vi "State Machine.vi"() -> ()   [LabVIEW 2020]
uses:
  enum control.ctl
  <vilib>/Utility/config.llb/NI_LVConfig.lvlib
panel:
  out "Ring":u16(ring)
  out "Time remaning":string
  out "numerator":dbl
  out "Duration of centrifugation":dbl
  out "Duration of rinsing":dbl
  out "Duration of washing":dbl
  out "Spin":dbl(slide) scale=0.0..1200.0
  out "Temperature":dbl(slide) scale=0.0..100.0
  out "Program 4":string
  out "Program 3":string
  out "Program 2":string
  out "Program 1":string
  in  "Stop Button":bool
  out "Lock Button":bool
  in  "Play Button":bool
  in  "Program":u32(knob) max=3 scale=0.0..3.0
  out "Centrifugation":bool
  out "Rinsing":bool
  out "Washing":bool
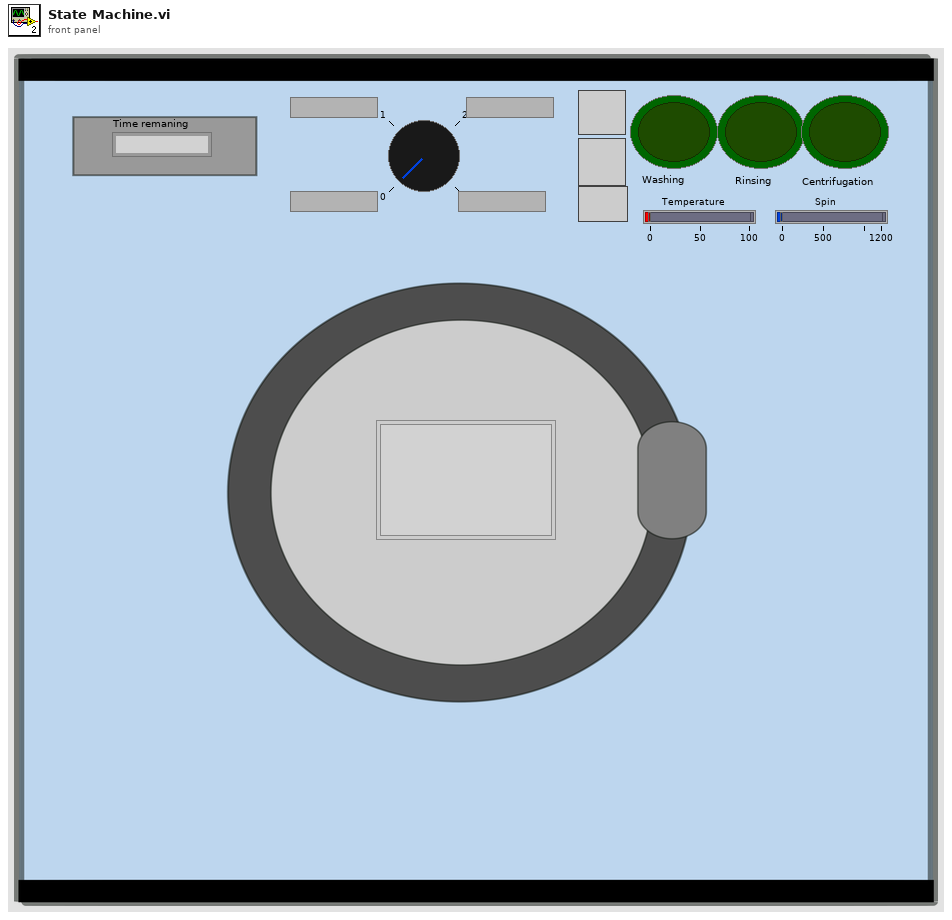
[diagram p1: front panel]
types:
  T1 = cluster{"Results":u32[], "Results":u32[], "Results":u32[], "Results":u32[]}
  T2 = typedef "enum control.ctl" = enum16{"Init", "Which program", "Block", "Washing", "Rinsing", "Centrifugation", "Unblock", "End"}
  T3 = enum8{"Enabled", "Disabled", "Disabled and Grayed Out"}
  T4 = typedef "NI_LVConfig.lvlib/Config Data RefNum.ctl" = refnum<k1>
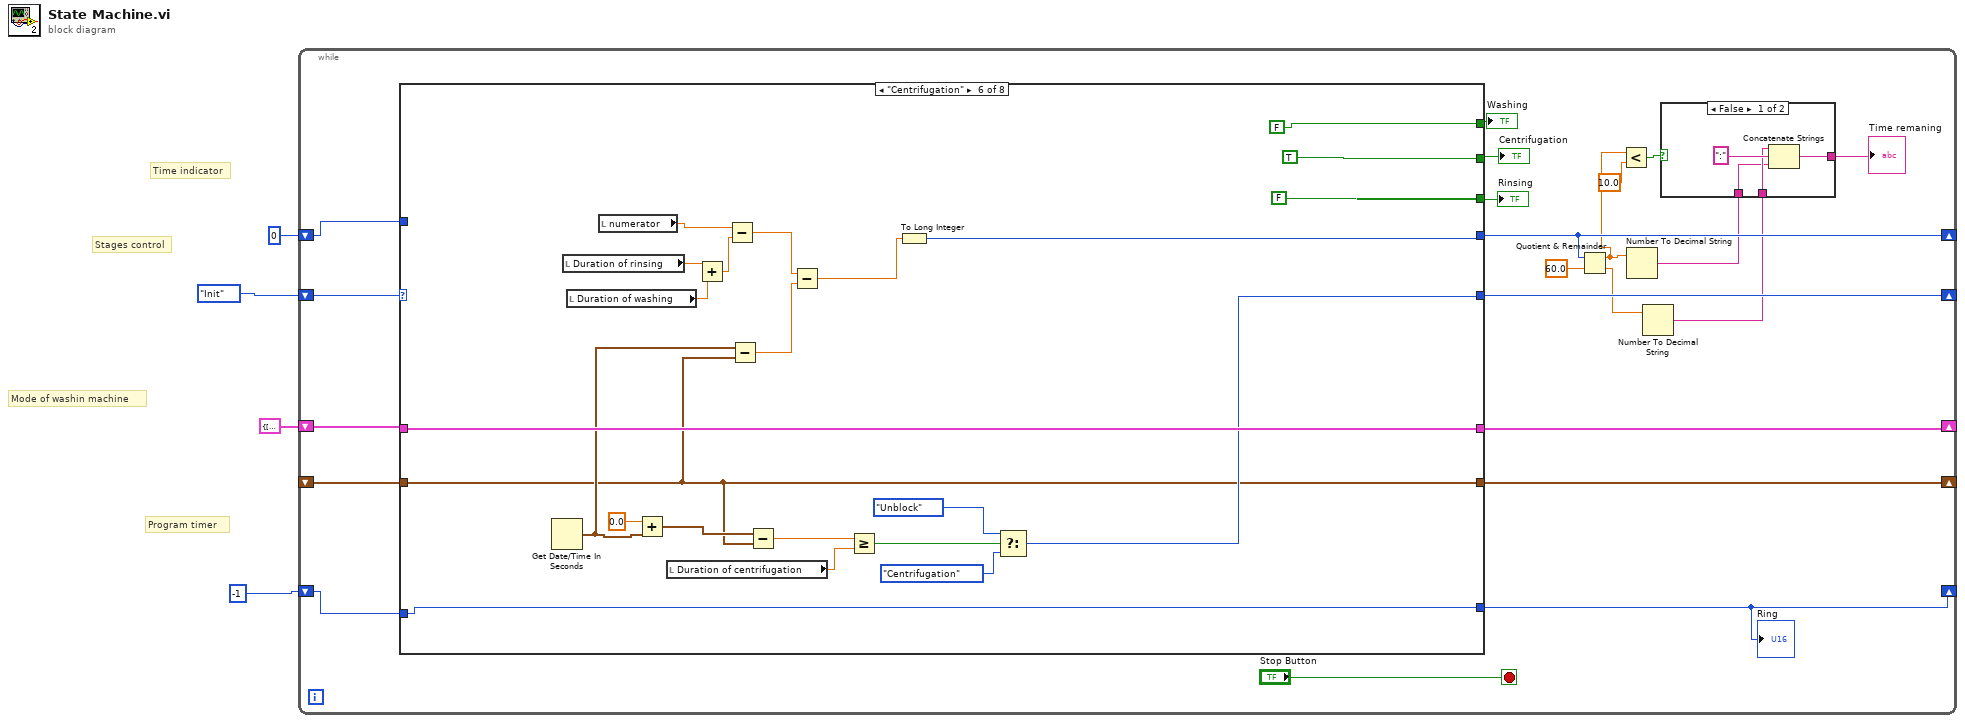
[diagram p0: block diagram]
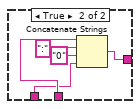
[diagram p2: hidden frame]
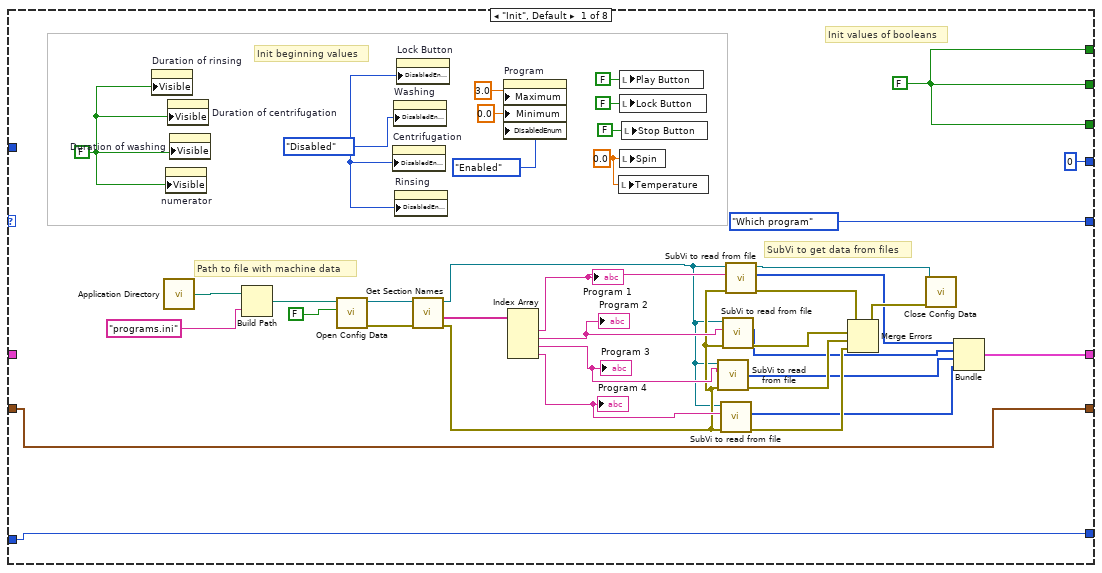
[diagram p3: hidden frame]
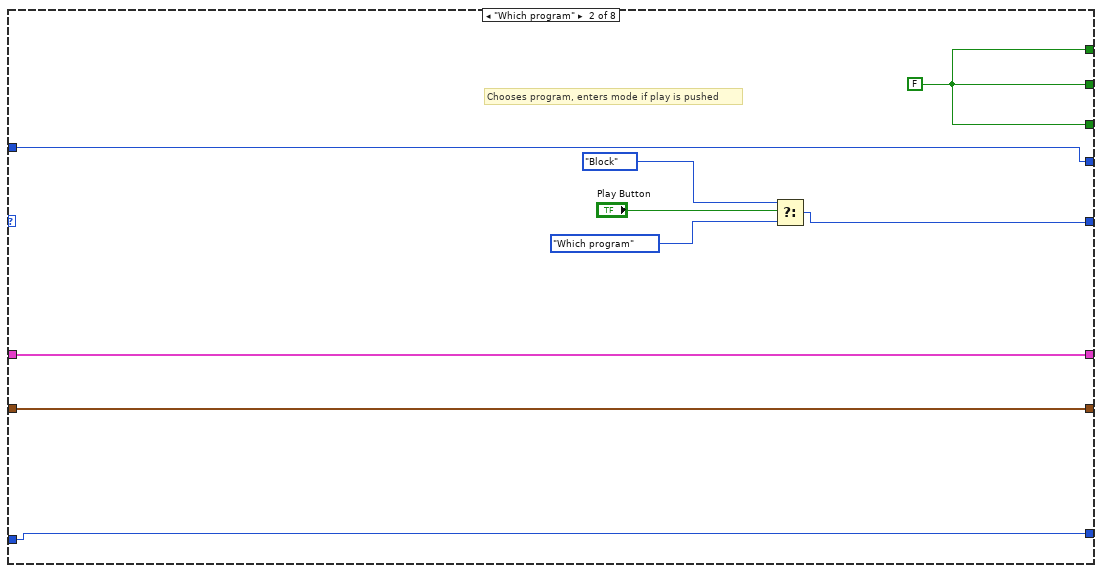
[diagram p4: hidden frame]
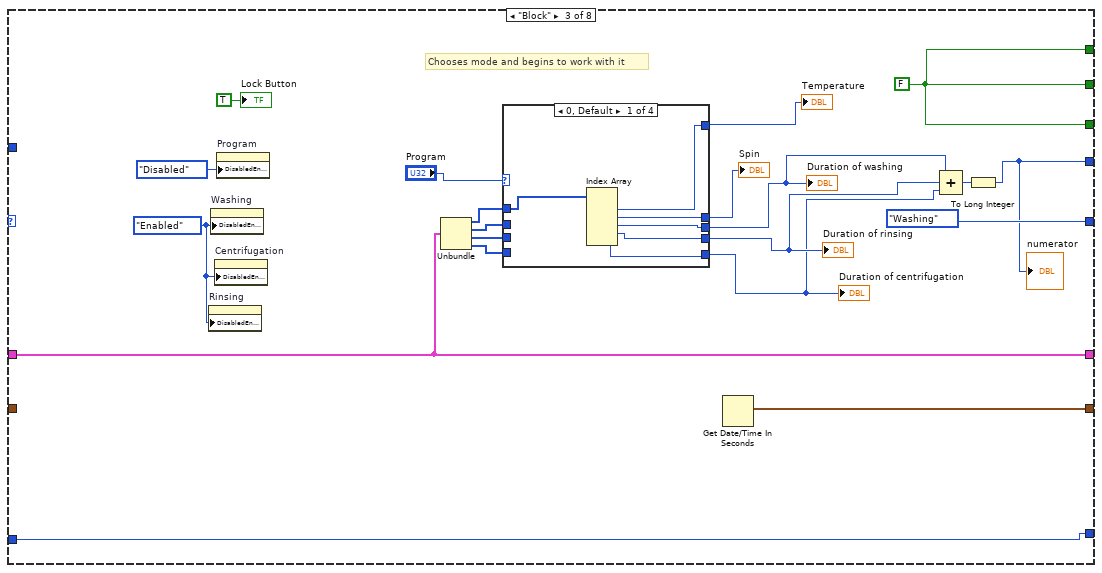
[diagram p5: hidden frame]
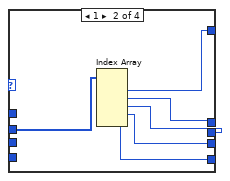
[diagram p6: hidden frame]
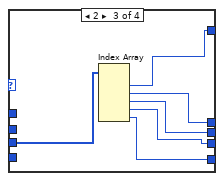
[diagram p7: hidden frame]
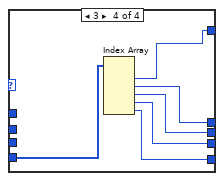
[diagram p8: hidden frame]
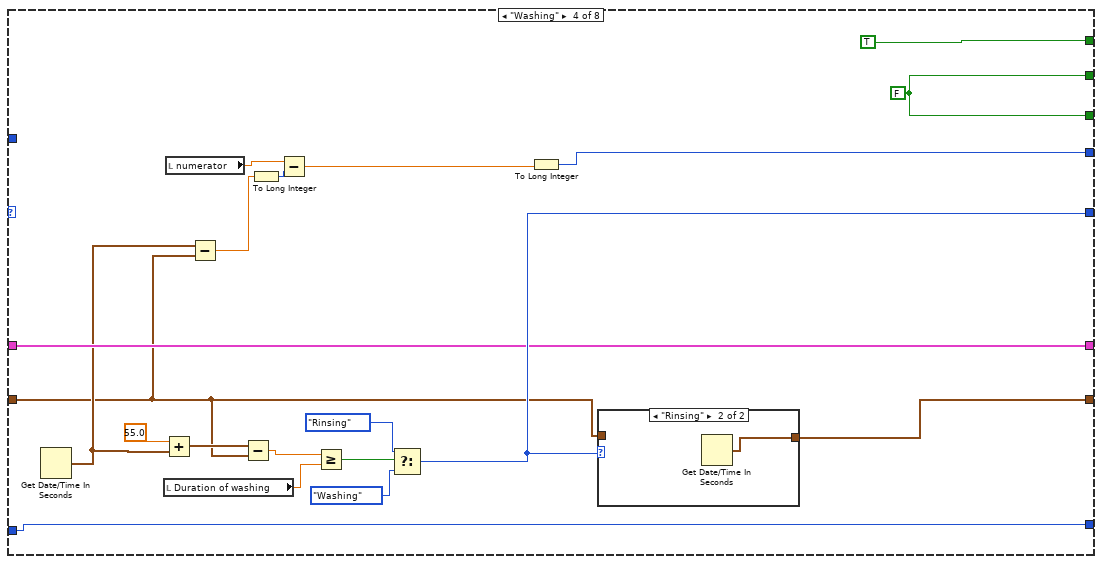
[diagram p9: hidden frame]
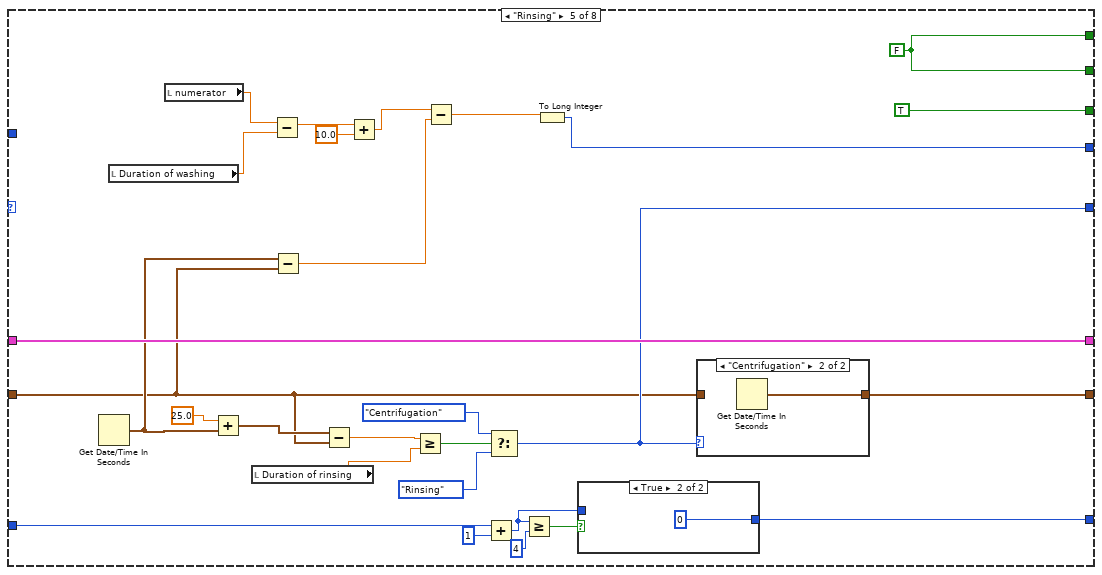
[diagram p11: hidden frame]
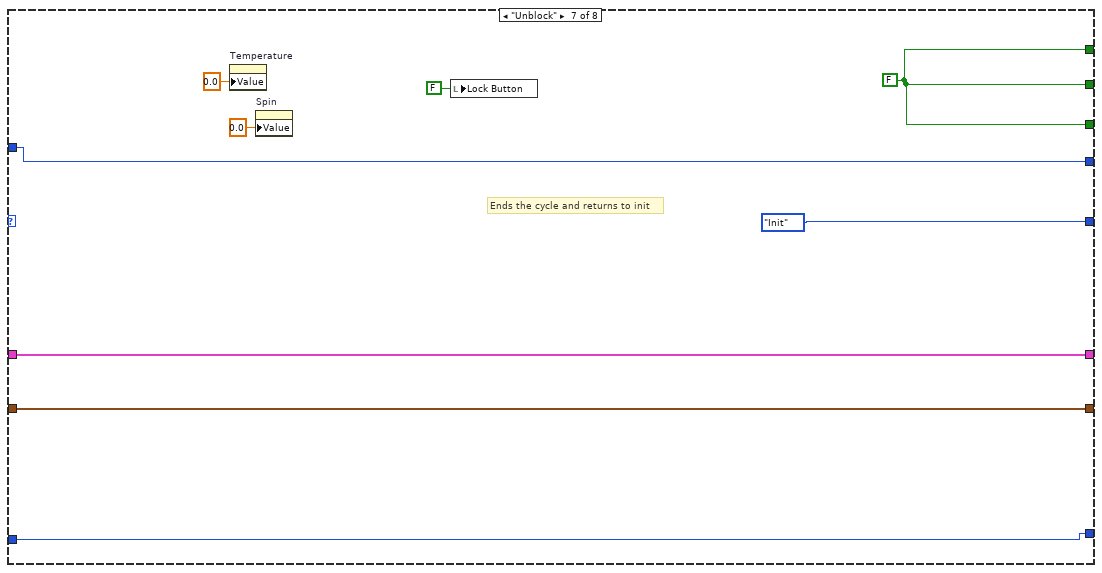
[diagram p14: hidden frame]
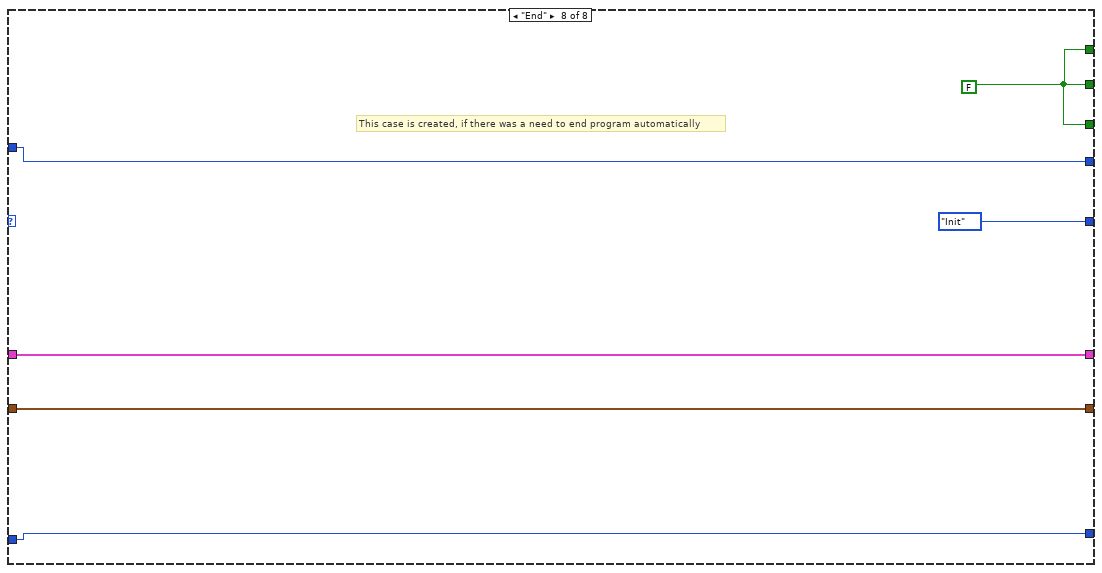
[diagram p15: hidden frame]
diagram:
  # "Mode of washin machine"
  # "Program timer"
  # "Time indicator"
  # "Stages control"
  n1 = while {
    shift-right: [w24] -> _
    shift-left: enum_control."Init" -> [w26]
    shift-right: [w20] -> _
    shift-left: T1 {"Results"=[], "Results"=[], "Results"=[], "Results"=[]} -> [w19]
    shift-right: [w18] -> _
    shift-left: _ -> [w17]
    shift-right: [w14] -> _
    shift-left: 0 -> [w16]
    shift-right: [w11] -> _
    shift-left: -1 -> [w12]
    stop <- "Stop Button" stop-if-true
    n2 = case shown="\"Centrifugation\"" w26 {
      tunnel: [enum_control."Which program" w79 enum_control."Washing" w140 w168 w194 enum_control."Init" enum_control."Init"] -> w24
      tunnel: [w65 w82 w101 TRUE ("Play Button") w176 FALSE ("Play Button") w211 w218] -> w23
      tunnel: [w65 w82 w101 w145 w176 TRUE ("Play Button") w211 w218] -> w22
      tunnel: [w65 w82 w101 w145 TRUE ("Play Button") FALSE ("Play Button") w211 w218] -> w21
      tunnel: [w41 w81 w96 w138 w174 w200 w210 w216] -> w20
      tunnel: w19 -> [_ w81 w96 w138 w174 w200 w210 w216]
      tunnel: [w40 w76 w91 w139 w167 w185 w209 w215] -> w18
      tunnel: w17 -> [w40 w76 _ w128 w161 w185 w209 w215]
      tunnel: [0 w75 w84 w137 w164 w192 w207 w217] -> w14
      tunnel: w16 -> [_ w75 _ _ _ _ w207 w217]
      tunnel: w12 -> [w37 w74 w83 w127 w154 w181 w206 w213]
      tunnel: [w37 w74 w83 w127 w150 w181 w206 w213] -> w11
      frame "Init", Default {
        w36 = FALSE ("Visible")
        w65 = FALSE ("Play Button")
        w67 = T3."Disabled" ("Disabled")
        w70 = 0.0 ("Spin")
        # "Init values of booleans"
        # "SubVi to get data from files"
        # "Init beginning values"
        # "Path to file with machine data"
        n3 = property on="Duration of rinsing" class="DigNum (strict)"("Visible"=w36) -> ()  [unwired: 2 in, 2 out]
        n4 = call <vilib>:"Application Directory.vi"() -> ("Application Directory"=w64:path)
        n5 = property on="numerator" class="DigNum (strict)"("Visible"=w36) -> ()  [unwired: 2 in, 2 out]
        n6 = property on="Duration of centrifugation" class="DigNum (strict)"("Visible"=w36) -> ()  [unwired: 2 in, 2 out]
        n7 = property on="Duration of washing" class="DigNum (strict)"("Visible"=w36) -> ()  [unwired: 2 in, 2 out]
        n8 = Build Path(base path=w64, name or relative path="programs.ini") -> (appended path=w63:path)
        n9 = call <vilib>:"Open Config Data.vi"("create file if necessary (T)"=FALSE, "configuration file path"=w63) -> ("error out"=w61:errorcluster, "refnum"=w60:T4)  [unwired: 7 in, 1 out]
        n10 = property on="Centrifugation" class="Bool (strict)"("DisabledEnum"=w67) -> ()  [unwired: 2 in, 2 out]
        n11 = property on="Washing" class="Bool (strict)"("DisabledEnum"=w67) -> ()  [unwired: 2 in, 2 out]
        n12 = property on="Rinsing" class="Bool (strict)"("DisabledEnum"=w67) -> ()  [unwired: 2 in, 2 out]
        n13 = property on="Lock Button" class="Bool"("DisabledEnum"=w67) -> ()  [unwired: 2 in, 2 out]
        n14 = call <vilib>:"Get Section Names.vi"("error in (no error)"=w61, "refnum"=w60) -> ("error out"=w54:errorcluster, "section names"=w59:string[], "refnum out"=w53:T4)  [unwired: 7 in]
        n15 = property on="Program" class="Knob (strict)"("Maximum"=3.0 ("Data Entry Limits:Maximum"), "Minimum"=0.0 ("Data Entry Limits:Minimum"), "DisabledEnum"=T3."Enabled" ("Disabled")) -> ()  [unwired: 2 in, 2 out]
        n16 = Index Array(array=w59) -> (element #1=w58:string, element #2=w57:string, element #3=w56:string, element #4=w55:string)  [unwired: 4 in]
        "Program 1" <- w58
        "Program 2" <- w57
        "Program 3" <- w56
        "Program 4" <- w55
        n17 = local write "Temperature"(w70) -> ()
        n18 = local write "Play Button"(FALSE ("Play Button")) -> ()
        n19 = local write "Lock Button"(FALSE ("Lock Button")) -> ()
        n20 = local write "Spin"(w70) -> ()
        n21 = local write "Stop Button"(FALSE ("Stop Button")) -> ()
        n22 = call "SubVi to read from file.vi"("error in (no error)"=w54, "section"=w56, "Refnum in"=w53) -> ("error out"=w50:errorcluster, "Results"=w43:u32[])  [unwired: 6 in, 1 out]
        n23 = call "SubVi to read from file.vi"("error in (no error)"=w54, "section"=w55, "Refnum in"=w53) -> ("error out"=w49:errorcluster, "Results"=w42:u32[])  [unwired: 6 in, 1 out]
        n24 = call "SubVi to read from file.vi"("error in (no error)"=w54, "section"=w57, "Refnum in"=w53) -> ("error out"=w51:errorcluster, "Results"=w44:u32[])  [unwired: 6 in, 1 out]
        n25 = call "SubVi to read from file.vi"("error in (no error)"=w54, "section"=w58, "Refnum in"=w53) -> ("error out"=w52:errorcluster, "Results"=w45:u32[], "Refnum out"=w47:T4)  [unwired: 6 in]
        n26 = Merge Errors(w52, w51, w50, w49) -> (w48:errorcluster)
        n27 = call <vilib>:"Close Config Data.vi"("error in (no error)"=w48, "refnum"=w47) -> ()  [unwired: 8 in, 2 out]
        n28 = Bundle("Results"=w45, "Results"=w44, "Results"=w43, "Results"=w42) -> (w41:T1)  [unwired: 1 in]
      }
      frame "Which program" {
        w82 = FALSE ("Play Button")
        # "Chooses program, enters mode if play is pushed"
        n29 = Select(t=enum_control."Block", s="Play Button", f=enum_control."Which program") -> (s? t:f=w79:T2)
      }
      frame "Block" {
        w98 = T3."Enabled" ("Disabled")
        w101 = FALSE ("Play Button")
        # "Chooses mode and begins to work with it"
        n30 = property on="Rinsing" class="Bool (strict)"("DisabledEnum"=w98) -> ()  [unwired: 2 in, 2 out]
        n31 = property on="Washing" class="Bool (strict)"("DisabledEnum"=w98) -> ()  [unwired: 2 in, 2 out]
        n32 = property on="Centrifugation" class="Bool (strict)"("DisabledEnum"=w98) -> ()  [unwired: 2 in, 2 out]
        n33 = property on="Program" class="Knob (strict)"("DisabledEnum"=T3."Disabled" ("Disabled")) -> ()  [unwired: 2 in, 2 out]
        n34 = Unbundle(w96) -> ("Results"=w95:u32[], "Results"=w94:u32[], "Results"=w93:u32[], "Results"=w92:u32[])
        n35 = case shown="0, Default" "Program" {
          tunnel: w95 -> [w108 _ _ _]
          tunnel: w94 -> [_ w114 _ _]
          tunnel: w93 -> [_ _ w120 _]
          tunnel: w92 -> [_ _ _ w126]
          tunnel: [w107 w113 w119 w125] -> w89
          tunnel: [w106 w112 w118 w124] -> w90
          tunnel: [w105 w111 w117 w123] -> w88
          tunnel: [w104 w110 w116 w122] -> w87
          tunnel: [w103 w109 w115 w121] -> w86
          frame 0, Default {
            n36 = Index Array(array=w108) -> (element #1=w107:u32, element #2=w106:u32, element #3=w105:u32, element #4=w104:u32, element #5=w103:u32)  [unwired: 5 in]
          }
          frame 1 {
            n37 = Index Array(array=w114) -> (element #1=w113:u32, element #2=w112:u32, element #3=w111:u32, element #4=w110:u32, element #5=w109:u32)  [unwired: 5 in]
          }
          frame 2 {
            n38 = Index Array(array=w120) -> (element #1=w119:u32, element #2=w118:u32, element #3=w117:u32, element #4=w116:u32, element #5=w115:u32)  [unwired: 5 in]
          }
          frame 3 {
            n39 = Index Array(array=w126) -> (element #1=w125:u32, element #2=w124:u32, element #3=w123:u32, element #4=w122:u32, element #5=w121:u32)  [unwired: 5 in]
          }
        }
        "Spin" <- w90
        "Temperature" <- w89
        "Duration of washing" <- w88
        "Duration of rinsing" <- w87
        "Duration of centrifugation" <- w86
        n40 = Get Date/Time In Seconds() -> (seconds since 1Jan1904=w91:timestamp)
        n41 = Compound Arithmetic op=ADD(w88, w87, w86) -> (w85:u32)
        n42 = To Long Integer(number=w85) -> (32bit integer=w84:i32)
        "numerator" <- w84
        "Lock Button" <- TRUE ("Lock Button")
      }
      frame "Washing" {
        w145 = FALSE ("Play Button")
        n43 = Get Date/Time In Seconds() -> (seconds since 1Jan1904=w129:timestamp)
        n44 = Add(x=55.0, y=w129) -> (x+y=w130:timestamp)
        n45 = local read "Duration of washing"() -> (w136:dbl)
        n46 = local read "numerator"() -> (w133:dbl)
        n47 = Subtract(x=w129, y=w128) -> (x-y=w131:dbl)
        n48 = Subtract(x=w130, y=w128) -> (x-y=w132:dbl)
        n49 = To Long Integer(number=w131) -> (32bit integer=w135:i32)
        n50 = Subtract(x=w133, y=w135) -> (x-y=w134:dbl)
        n51 = Greater Or Equal?(x=w132, y=w136) -> (x >= y?=w143:bool)
        n52 = Select(t=enum_control."Rinsing", s=w143, f=enum_control."Washing") -> (s? t:f=w140:T2)
        n53 = To Long Integer(number=w134) -> (32bit integer=w137:i32)
        n54 = case shown="\"Rinsing\"" w140 {
          tunnel: w128 -> [w147 _]
          tunnel: [w147 w148] -> w139
          frame "Washing", Default {
          }
          frame "Rinsing" {
            n55 = Get Date/Time In Seconds() -> (seconds since 1Jan1904=w148:timestamp)
          }
        }
      }
      frame "Rinsing" {
        w176 = FALSE ("Play Button")
        n56 = Get Date/Time In Seconds() -> (seconds since 1Jan1904=w162:timestamp)
        n57 = local read "Duration of washing"() -> (w158:dbl)
        n58 = local read "numerator"() -> (w159:dbl)
        n59 = Add(x=25.0, y=w162) -> (x+y=w172:timestamp)
        n60 = local read "Duration of rinsing"() -> (w163:dbl)
        n61 = Subtract(x=w159, y=w158) -> (x-y=w156:dbl)
        n62 = Subtract(x=w162, y=w161) -> (x-y=w160:dbl)
        n63 = Subtract(x=w172, y=w161) -> (x-y=w165:dbl)
        n64 = Add(x=w156, y=10.0) -> (x+y=w157:dbl)
        n65 = Greater Or Equal?(x=w165, y=w163) -> (x >= y?=w171:bool)
        n66 = Subtract(x=w157, y=w160) -> (x-y=w166:dbl)
        n67 = Add(x=w154, y=1) -> (x+y=w149:i32)
        n68 = Select(t=enum_control."Centrifugation", s=w171, f=enum_control."Rinsing") -> (s? t:f=w168:T2)
        n69 = Greater Or Equal?(x=w149, y=4) -> (x >= y?=w151:bool)
        n70 = To Long Integer(number=w166) -> (32bit integer=w164:i32)
        n71 = case shown="True" w151 {
          tunnel: [w177 0] -> w150
          tunnel: w149 -> [w177 _]
          frame False {
          }
          frame True {
          }
        }
        n72 = case shown="\"Centrifugation\"" w168 {
          tunnel: w161 -> [w179 _]
          tunnel: [w179 w180] -> w167
          frame "Rinsing", Default {
          }
          frame "Centrifugation" {
            n73 = Get Date/Time In Seconds() -> (seconds since 1Jan1904=w180:timestamp)
          }
        }
      }
      frame "Centrifugation" {
        n74 = Get Date/Time In Seconds() -> (seconds since 1Jan1904=w186:timestamp)
        n75 = local read "Duration of rinsing"() -> (w189:dbl)
        n76 = local read "Duration of washing"() -> (w188:dbl)
        n77 = local read "numerator"() -> (w190:dbl)
        n78 = Add(x=0.0, y=w186) -> (x+y=w198:timestamp)
        n79 = local read "Duration of centrifugation"() -> (w191:dbl)
        n80 = Add(x=w189, y=w188) -> (x+y=w187:dbl)
        n81 = Subtract(x=w190, y=w187) -> (x-y=w184:dbl)
        n82 = Subtract(x=w186, y=w185) -> (x-y=w183:dbl)
        n83 = Subtract(x=w198, y=w185) -> (x-y=w193:dbl)
        n84 = Subtract(x=w184, y=w183) -> (x-y=w182:dbl)
        n85 = Greater Or Equal?(x=w193, y=w191) -> (x >= y?=w195:bool)
        n86 = To Long Integer(number=w182) -> (32bit integer=w192:i32)
        n87 = Select(t=enum_control."Unblock", s=w195, f=enum_control."Centrifugation") -> (s? t:f=w194:T2)
      }
      frame "Unblock" {
        w211 = FALSE ("Play Button")
        # "Ends the cycle and returns to init"
        n88 = property on="Temperature" class="Slide (strict)"("Value"=0.0 ("Temperature")) -> ()  [unwired: 2 in, 2 out]
        n89 = property on="Spin" class="Slide (strict)"("Value"=0.0 ("Spin")) -> ()  [unwired: 2 in, 2 out]
        n90 = local write "Lock Button"(FALSE ("Lock Button")) -> ()
      }
      frame "End" {
        w218 = FALSE
        # "This case is created, if there was a need to end program automatically"
      }
    }
    "Washing" <- w23
    "Centrifugation" <- w22
    "Rinsing" <- w21
    "Ring" <- w11
    n91 = Quotient & Remainder(x=w14, y=60.0) -> (x-y*floor(x/y)=w10:dbl, floor(x/y)=w13:dbl)
    n92 = Less?(x=w10, y=10.0) -> (x < y?=w8:bool)
    n93 = Number To Decimal String(number=w10) -> (decimal integer string=w7:string)  [unwired: 1 in]
    n94 = Number To Decimal String(number=w13) -> (decimal integer string=w6:string)  [unwired: 1 in]
    n95 = case shown="False" w8 {
      tunnel: w7 -> [w27 w32]
      tunnel: w6 -> [w28 w35]
      tunnel: [w29 w31] -> w5
      frame False {
        n96 = Concatenate Strings(w28, ":" ("string"), w27) -> (w29:string)
      }
      frame True {
        n97 = Concatenate Strings(w35, ":" ("string"), "0" ("string"), w32) -> (w31:string)
      }
    }
    "Time remaning" <- w5
  }
